vi "Alpha Ver 1.3.vi"() -> ()   [LabVIEW 2015]
uses:
  <instrlib>/Keithley 622x LV 2009/Configure/Source/Typedefs/KE622x -- Current Range.ctl
  <instrlib>/Keithley 622x LV 2009/Configure/Source/Typedefs/KE622x -- Current Ranges.ctl
  <instrlib>/Keithley 622x LV 2009/Typedefs/KE622x -- On Off Control.ctl
  <instrlib>/Keithley 622x LV 2009/Utility/Typedefs/KE622x -- Instrument Type.ctl
  <instrlib>/Keithley 622x LV 2009/Configure/Source/Typedefs/KE622x -- Voltage Limit.ctl
  <instrlib>/Keithley 2000/Public/Configure/Configure DC Volts.vi
  <userlib>/LV-Link3/PolySubVIs/DtCreateAinChan.vi
  <userlib>/LV-Link3/PolySubVIs/DtOLReadMultipleSingle.vi
  <instrlib>/Keithley 2000/Keithley 2000.lvlib
  <instrlib>/Keithley 622x LV 2009/Keithley 622x.lvlib
panel:
  in  "Lock-In, Y":dbl=1.0
  in  "Lock-In, X":dbl=1.0
  in  "DAQ A4":dbl=1.0
  in  "DAQ A3":dbl=1.0
  in  "DAQ A2":dbl=1.0
  in  "DAQ A1":dbl=1.0
  in  "DAQ A0":dbl=1.0
  in  "2000":dbl=1.0
  in  "Current":dbl=1000.0
  in  "Display Type 3":u16(ring)=3 items=["X %", "Y %", "X Calibrated", "Y Calibrated", "Mag %", "Mag Calibrated", "Phase Degrees", "Ratio", "ADC 1", "ADC 2", "ADC 3", "ADC 4 ", "Noise %", "Noise Calibrated", "Ref Frequency", "", ""]
  in  "Display Type 2":u16(ring)=2 items=["X %", "Y %", "X Calibrated", "Y Calibrated", "Mag %", "Mag Calibrated", "Phase Degrees", "Ratio", "ADC 1", "ADC 2", "ADC 3", "ADC 4 ", "Noise %", "Noise Calibrated", "Ref Frequency", "", ""]
  out "Units 3":string
  out "Display 3":dbl format="%.3f"
  out "Units 2":string
  out "Display 2":dbl format="%.3f"
  out "DAQ A4":dbl format="%#_13g"
  out "DAQ_clust":T1
  out "DAQ A3":dbl format="%#_13g"
  out "DAQ A2":dbl format="%#_13g"
  out "DAQ A1":dbl format="%#_13g"
  out "Real stop cur":dbl format="%#_13g"
  out "Real start cur":dbl format="%#_13g"
  in  "Stop cur prefix":u16(ring)=2
  in  "Start cur prefix":u16(ring)=2
  out "MULTIPLE GRAPHS":cluster{dbl[], dbl[]}[](graph)
  in  "X-Axis":T2(ring)
  in  "Range":u8(ring)=20 items=["100nV", "200nV", "500nV", "1µV", "2µV", "5µV", "10µV", "20µV", "50µV", "100µV", "200µV", "500µV", "1mV", "2mV", "5mV", "10mV", "20mV", "50mV", "100mV", "200mV", "500mV", "1V"]
  in  "Display Type copy":u16(ring)=3 items=["X %", "Y %", "X Calibrated", "Y Calibrated", "Mag %", "Mag Calibrated", "Phase Degrees", "Ratio", "ADC 1", "ADC 2", "ADC 3", "ADC 4 ", "Noise %", "Noise Calibrated", "Ref Frequency", "", ""]
  out "Units copy":string
  out "Display copy":dbl format="%.3f"
  out "Overload":bool
  out "Display":dbl format="%.3f"
  out "Units":string
  in  "Display Type":u16(ring)=2 items=["X %", "Y %", "X Calibrated", "Y Calibrated", "Mag %", "Mag Calibrated", "Phase Degrees", "Ratio", "ADC 1", "ADC 2", "ADC 3", "ADC 4 ", "Noise %", "Noise Calibrated", "Ref Frequency", "", ""]
  in  "Time Constant":u16(ring) items=["MIN", "1ms", "3ms", "10ms", "30ms", "100ms", "300ms", "1s", "3s", "10s", "30s", "100s", "300s"]
  in  "Slope":u8(ring) items=["6db/octave", "12dB/octave"]
  in  "Dynamic Reserve":u16(ring) items=["High Stability", "Normal", "High Reserve"]
  in  "Auto Sensitivity":bool
  in  "Auto Measure":bool
  out "6221_error_out":errorcluster
  out "2000_error_out":errorcluster
  out "5110_error_out":errorcluster
  out "Input Mode":i32(ring) items=[" Voltage Input (A or A-B) ", "Current Input 10E6 V/A", "Current Input 10E8 V/A"]
  out "5110":refnum<visa-resource-name>
  in  "GPIB Address":i8=11 min=1 max=32 step=1
  out "DAQ A0":dbl format="%#_13g"
  out "2000":dbl format="%#_13g"
  in  "Device":string(combo)
  in  "Number \nof points":i32
  in  "Folder\nprename":string
  out "TIME GRAPH":cluster{dbl[], dbl[]}[](graph)
  out "T0":u32
  out "LIMIT":bool
  out "LIMIT":bool
  out "Error Code":string
  in  "Comments":string
  out "file":refnum<file>
  out "2000":refnum<visa-resource-name>
  out "6221":refnum<visa-resource-name>
  out "Step  (A)":dbl=5e-05 format="%#_3p"
  in  "Stop\ncurrent (A)":dbl=2.0 format="%#_6p"
  in  "Start \ncurrent (A)":dbl=1.0 format="%#_6p"
  in  "Check For SCPI Errors? (T)":bool=TRUE
  out "Interlock Tripped?":bool
  out "Compliance?":bool
  in  "Turn Off Output \nIf Compliance?":bool=TRUE
  in  "Turning ON/OFF\ncurrent output":T3=enum."On"
  in  "Range Selection":T4={"Auto Range?"=TRUE, "Man / Selected\nRange"=enum."2nA"}
  # "FILE CONFIGURATION"
  # "ADMIN PANEL"
  # "KEITHLEY 6221 CONFIGURATION (ADMIN ONLY)"
  # "KEITHLEY DAQ CONFIGURATION (ADMIN ONLY)"
  # "PRINCETON LOCK-IN AMP (ADMIN ONLY)"
  # "I don't know what the hell it is,\njust don't touch it"
  # "SENSITIVITY"
  # "INPUT CONFIGURATION"
  # "READINGS"
  # "START, STOP, STEP, CONFIGURATION"
  # "IF ON"
  # "Output Channels Time - Constant \nSlope & Dynamic Reserve"
  # "Compliance = Limiting output voltage\nThis switch determines if we want to switch \noff the current output if wee exceed compliance"
  # "LOCK-IN READINGS"
  # "RIGHT DISPLAY"
  # "LEFT DISPLAY"
  # "There is a safe switch at \nthe back of the instrument \nThis indicator shows if it is on"
  # "You have hit a damn jackpot \nby exceeding the limited voltage\nCongrats"
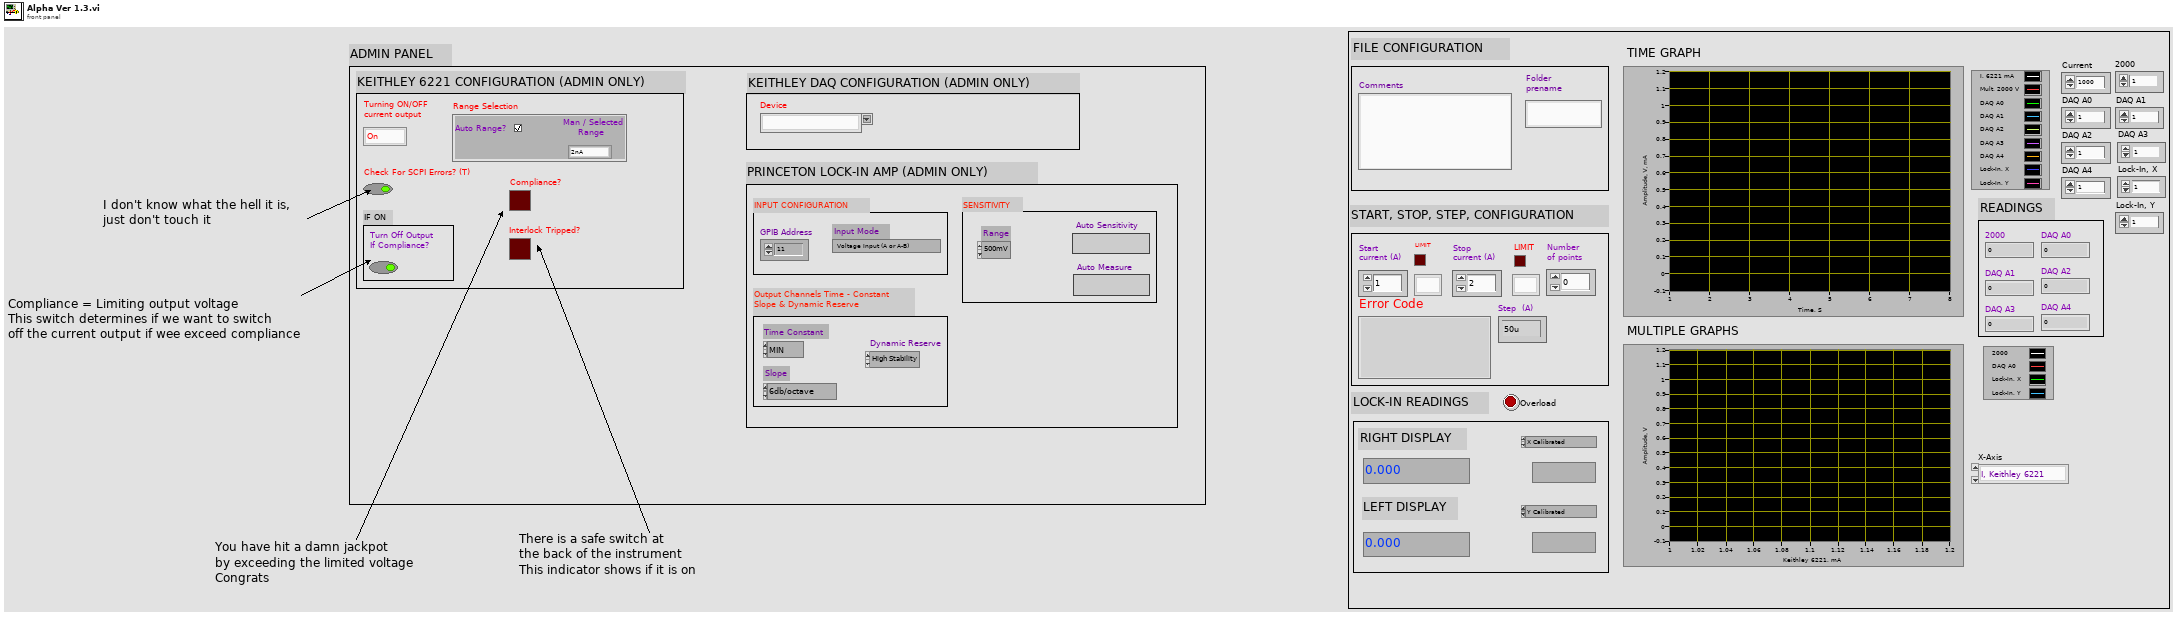
[diagram p1: front panel]
types:
  T1 = cluster{"Task out":i32, "Actual Number of Channels":u32, "error out":errorcluster}
  T2 = enum16{"I, Keithley 6221", "V, Keithley 2000", "V, Keithley DAQ A0", "V, Keithley DAQ A1", "V, Keithley DAQ A2", "V, Keithley DAQ A3", "V, Keithley DAQ A4", "V, Lock-In X", "V, Lock-In Y"}
  T3 = typedef "Keithley 622x.lvlib/KE622x -- On Off Control.ctl" = enum16{"Off", "On"}
  T4 = typedef "Keithley 622x.lvlib/KE622x -- Current Range.ctl" = cluster{"Auto Range?":bool, "Man / Selected\nRange":T5}
  T5 = typedef "Keithley 622x.lvlib/KE622x -- Current Ranges.ctl" = enum16{"2nA", "20nA", "200nA", "2uA", "20uA", "200uA", "2mA", "20mA", "100mA"}
  T6 = typedef "Keithley 622x.lvlib/KE622x -- Instrument Type.ctl" = enum16{"KE6220", "KE6221"}
  T7 = typedef "Keithley 622x.lvlib/KE622x -- Voltage Limit.ctl" = dbl
  T8 = cluster{"Task out":i32, "error out":errorcluster}
  T9 = cluster{dbl, dbl, dbl, dbl, dbl, "Measurement":dbl}
  T10 = cluster{dbl[], dbl[], dbl[], dbl[], dbl[], dbl[], dbl[], dbl[], dbl[], dbl[]}
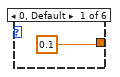
[diagram p2: hidden frame]
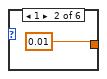
[diagram p3: hidden frame]
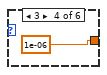
[diagram p4: hidden frame]
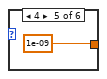
[diagram p5: hidden frame]
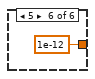
[diagram p6: hidden frame]
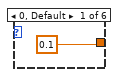
[diagram p7: hidden frame]
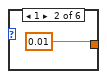
[diagram p8: hidden frame]
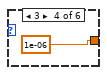
[diagram p9: hidden frame]
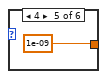
[diagram p10: hidden frame]
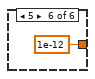
[diagram p11: hidden frame]
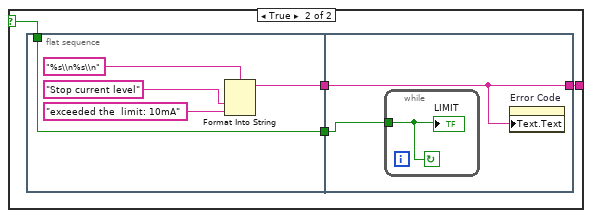
[diagram p12: hidden frame]
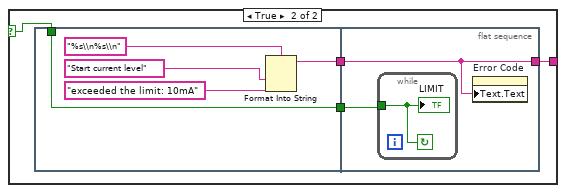
[diagram p13: hidden frame]
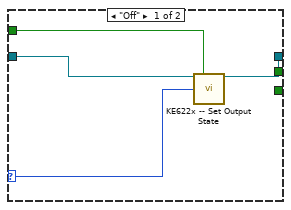
[diagram p14: hidden frame]
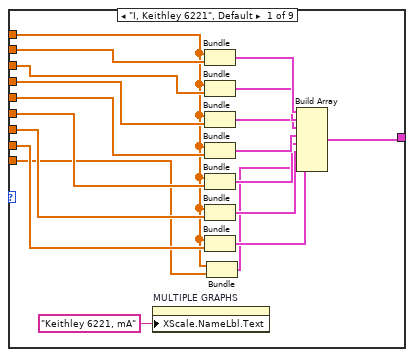
[diagram p15: hidden frame]
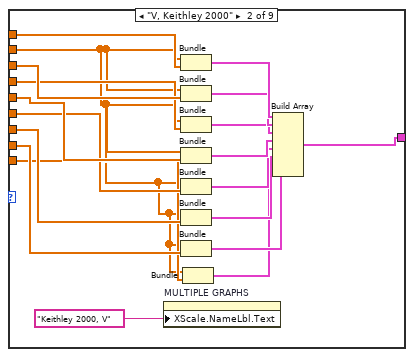
[diagram p16: hidden frame]
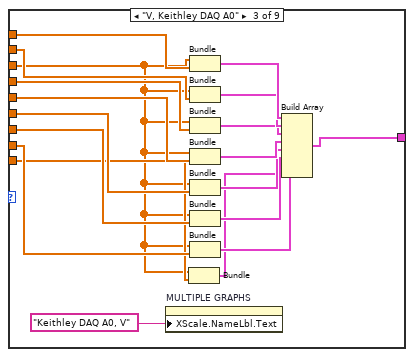
[diagram p17: hidden frame]
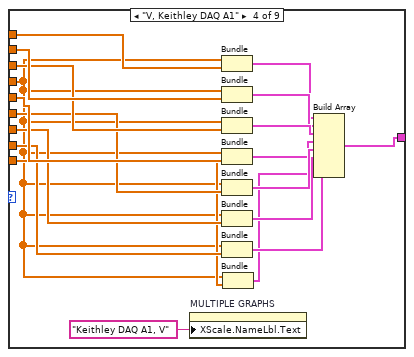
[diagram p18: hidden frame]
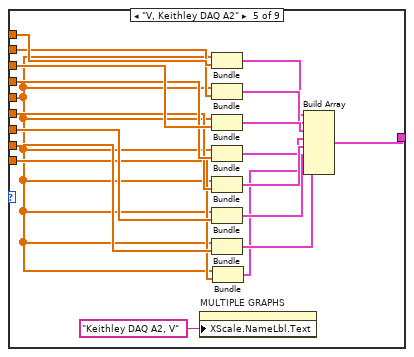
[diagram p19: hidden frame]
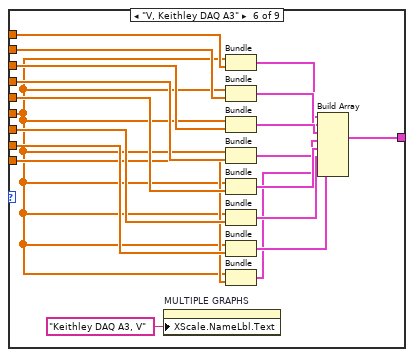
[diagram p20: hidden frame]
diagram:
  n1 = flat-sequence {
    tunnel: [w175] -> w7
    tunnel: [w174] -> w6
    tunnel: [w173] -> w5
    tunnel: [w172] -> w4
    tunnel: [w171] -> w3
    tunnel: [w170] -> w2
    tunnel: [w159] -> w1
    tunnel: w7 -> [w889]
    tunnel: w6 -> [w888]
    tunnel: w5 -> [w887]
    tunnel: w4 -> [w886]
    tunnel: w3 -> [w885]
    tunnel: w2 -> [w884]
    tunnel: w1 -> [w883]
    frame #0 {
      # "File configuration"
      # "Start, Stop, Step"
      # "Time Intit"
      # "Initializing instruments"
      n2 = flat-sequence {
        frame #0 {
          w16 = TRUE  # reset
          w15 = FALSE  # ID query
          # "Initialize Lock-In 5110"
          # "Initialize Keithley 2000"
          # "Initialize Keithley 6221"
          n3 = call <instrlib>:"Initialize.vi"("VISA resource name"=refnum<visa-resource-name> "KEITHLEY_MULTIMETER") -> ("VISA resource name out"=w20:refnum<visa-resource-name>)  [unwired: 17 in, 1 out]
          n4 = call <instrlib>:"Initialize.vi"("VISA resource name"=refnum<visa-resource-name> "KEITHLEY_DC_AC_CURRENT_SOURCE", "Error Queue Option"=enum16{"Clear Error Queue", "Error Query"}."Clear Error Queue", "Instrument Type"=KE622x_--_Instrument_Type."KE6221") -> ("VISA resource name out"=→"6221":refnum<visa-resource-name>, "error out"=→"6221_error_out":errorcluster)  [unwired: 11 in]
          n5 = call "SR51XX Initialize"("VISA session (for class)"=refnum<visa-resource-name> "LOCK_IN_5110_PRINCETON", "Interface"=FALSE, "ID query"=w15, "GPIB Address"="GPIB Address", "reset"=w16) -> ("VISA session"=→"5110":refnum<visa-resource-name>, "error out"=→"5110_error_out":errorcluster)  [unwired: 8 in, 1 out]
          n6 = call-poly <instrlib>:"Configure Measurement.vi"("VISA resource name"=w20) -> ("VISA resource name out"=→"2000":refnum<visa-resource-name>, "error out"=→"2000_error_out":errorcluster)  [unwired: 17 in]
        }
        frame #1 {
          # "Initialize Keithley DAQ \n(getting board name)"
          n7 = call <userlib>:"DtOLGetBoardNames.vi"() -> ("Number of boards"=w25:u32)  [unwired: 9 in, 2 out]
          n8 = Initialize Array("", w25) -> (w27:string[])
          n9 = for {
            N: w25 -> [_]
            shift-right: [w33] -> w30
            shift-left: w27 -> [w34]
            i -> [w32]
            n10 = Add(x=1, y=w32) -> (x+y=w36:i32)
            n11 = call <userlib>:"DtOLGetBoardNames.vi"("Select Board"=w36) -> ("Board Name"=w31:string)  [unwired: 8 in, 2 out]
            n12 = Replace Array Subset(array=w34, new element=w31, index=w32) -> (w33:string[])
          }
          n13 = Index Array(array=w30, index=0) -> (element=w29:string)
          n14 = property on="Device" class="CmbBox"("Strings[]"=w30, "Value"=w29) -> ()  [unwired: 2 in, 2 out]
        }
        frame #2 {
          # "Calculating steps by number\nof points"
          # "Putting in a loop \ninstead of \"STOP\""
          n15 = local read "Real stop cur"() -> (w53:dbl)
          n16 = local read "Real start cur"() -> (w54:dbl)
          n17 = case shown="2" "Start cur prefix" {
            tunnel: [0.1 0.01 0.001 1e-06 1e-09 1e-12] -> w42
            frame 0, Default {
            }
            frame 1 {
            }
            frame 2 {
            }
            frame 3 {
            }
            frame 4 {
            }
            frame 5 {
            }
          }
          n18 = case shown="2" "Stop cur prefix" {
            tunnel: [0.1 0.01 0.001 1e-06 1e-09 1e-12] -> w40
            frame 0, Default {
            }
            frame 1 {
            }
            frame 2 {
            }
            frame 3 {
            }
            frame 4 {
            }
            frame 5 {
            }
          }
          n19 = Subtract(x=w53, y=w54) -> (x-y=w56:dbl)
          n20 = Multiply(x=w42, y="Start \ncurrent (A)") -> (x*y=w38:dbl)
          "Real start cur" <- w38
          n21 = Divide(x=w56, y="Number \nof points") -> (x/y=→"Step  (A)":dbl)
          n22 = Multiply(x=w40, y="Stop\ncurrent (A)") -> (x*y=w37:dbl)
          "Real stop cur" <- w37
          n23 = Greater?(x=w37, y=T7 0.01) -> (0:w48:bool)
          n24 = Greater?(x=w38, y=T7 0.01) -> (0:w47:bool)
          n25 = case shown="False" w48 {
            selector: w48 -> [_ w72]
            tunnel: [w69 w75] -> w50
            frame False {
              n26 = Format Into String(format string="%s\\n", "Start current level is OK" ("false string")) -> (resulting string=w69:string)  [unwired: 2 in, 1 out]
            }
            frame True {
              n27 = flat-sequence {
                tunnel: [w77] -> w74
                tunnel: [w76] -> w73
                tunnel: w72 -> [w76]
                tunnel: [w81] -> w75
                tunnel: w74 -> [w81]
                tunnel: w73 -> [w82]
                frame #0 {
                  n28 = Format Into String(format string="%s\\n%s\\n", "Stop current level" ("String"), "exceeded the  limit: 10mA" ("input 2")) -> (resulting string=w77:string)  [unwired: 2 in, 1 out]
                }
                frame #1 {
                  n29 = while {
                    tunnel: w82 -> [w83]
                    stop <- w83 continue-if-true
                    "LIMIT" <- w83
                  }
                  n30 = property on="Error Code" class="Str"("Text.Text"=w81) -> ()  [unwired: 2 in, 2 out]
                }
              }
            }
          }
          n31 = case shown="False" w47 {
            selector: w47 -> [_ w88]
            tunnel: [w84 w90] -> w49
            frame False {
              n32 = Format Into String(format string="%s\\n", "Start current level is OK" ("false string")) -> (resulting string=w84:string)  [unwired: 2 in, 1 out]
            }
            frame True {
              n33 = flat-sequence {
                tunnel: [w92] -> w89
                tunnel: w88 -> [w91]
                tunnel: [w91] -> w87
                tunnel: [w96] -> w90
                tunnel: w89 -> [w96]
                tunnel: w87 -> [w97]
                frame #0 {
                  n34 = Format Into String(format string="%s\\n%s\\n", "Start current level" ("String"), "exceeded the limit: 10mA" ("input 2")) -> (resulting string=w92:string)  [unwired: 2 in, 1 out]
                }
                frame #1 {
                  n35 = while {
                    tunnel: w97 -> [w98]
                    stop <- w98 continue-if-true
                    "LIMIT" <- w98
                  }
                  n36 = property on="Error Code" class="Str"("Text.Text"=w96) -> ()  [unwired: 2 in, 2 out]
                }
              }
            }
          }
          n37 = Concatenate Strings(w49, w50) -> (→"Error Code":string)
        }
        frame #3 {
          n38 = flat-sequence {
            frame #0 {
              # "Creating folder&file"
              n39 = call "folder_creation.vi"("Name"="Folder\nprename") -> ("String"=w100:string)
              n40 = call "file_creation.vi"("String"=w100) -> ("refnum out"=→"file":refnum<file>)
            }
            frame #1 {
              # "Creating comments"
              n41 = local read "file"() -> (w102:refnum<file>)
              n42 = Format Into String(format string="# %s\\n", initial string=w102, "Comments") -> ()  [unwired: 1 in, 2 out]
            }
            frame #2 {
              # "Writing instr params"
              n43 = local read "5110"() -> (w110:refnum<visa-resource-name>)
              n44 = local read "Real stop cur"() -> (w108:dbl)
              n45 = local read "file"() -> (w105:refnum<file>)
              n46 = local read "Real start cur"() -> (w109:dbl)
              n47 = call "com_inst.vi"("Stop current"=w108, "Start current"=w109, "VISA session (for class)"=w110) -> ("concatenated string"=w106:string)
              n48 = Format Into String(format string="# %s\\n", initial string=w105, w106) -> ()  [unwired: 1 in, 2 out]
            }
            frame #3 {
              # "Adding headlines"
              n49 = local read "file"() -> (w122:refnum<file>)
              n50 = Format Into String(format string="# %-6s  %-12s %-12s %-14s %-12s %-14s %-12s %-12s %-14s%-14s\\n", initial string=w122, "t, s" ("input 3"), "2000, V" ("input 1"), "DAQ A0, V" ("input 2"), "DAQ A1, V" ("input 2"), "DAQ A2, V" ("input 2"), "DAQ A3, V" ("input 2"), "DAQ A4, V" ("input 2"), "5110_X, V" ("input 3"), "5110_Y, V " ("input 3"), "6221, A" ("input 3")) -> ()  [unwired: 1 in, 2 out]
            }
          }
        }
      }
      n51 = Tick Count (ms)() -> (millisecond timer value=→"T0":u32)
    }
    frame #1 {
      # "Configuring Keithley DAQ just before measuments"
      # "Configuring Keithley 6221 just before measuments"
      n52 = flat-sequence {
        tunnel: [w133] -> w123
        tunnel: [w151] -> _
        tunnel: [w153] -> _
        tunnel: w123 -> [w152]
        frame #0 {
          # "Current range \nselection check"
          # "Checking for compliance\nand interlock errors"
          n53 = local read "6221"() -> (w136:refnum<visa-resource-name>)
          n54 = call <instrlib>:"KE622x -- Set Current Range.vi"("Resource In"=w136, "Current Range In"="Range Selection", "Read Back Set Values? (T)"=FALSE) -> ("Resource Out (dupl)"=w141:refnum<visa-resource-name>)  [unwired: 10 in, 2 out]
          n55 = case shown="\"On\"" "Turning ON/OFF\ncurrent output" {
            selector: "Turning ON/OFF\ncurrent output" -> [w145 _]
            tunnel: [_ w149] -> w139
            tunnel: [_ w148] -> w140
            tunnel: "Check For SCPI Errors? (T)" -> [w144 _]
            tunnel: w141 -> [w142 w147]
            tunnel: [w143 w146] -> w133
            frame "Off" {
              n56 = call <instrlib>:"KE622x -- Set Output State.vi"("Resource In"=w142, "Check For SCPI Errors? (T)"=w144, "Output State"=w145) -> ("Resource Out (dupl)"=w143:refnum<visa-resource-name>)  [unwired: 11 in, 1 out]
            }
            frame "On" {
              n57 = call <instrlib>:"KE622x -- Turn Output On And Check For Errors.vi"("Resource In"=w147, "Turn Off Output If Compliance?"="Turn Off Output \nIf Compliance?") -> ("Resource Out (dupl)"=w146:refnum<visa-resource-name>, "Interlock Tripped?"=w149:bool, "Compliance?"=w148:bool)  [unwired: 10 in, 1 out]
            }
          }
          "Interlock Tripped?" <- w139
          "Compliance?" <- w140
        }
        frame #1 {
          # "Setting start current"
          n58 = local read "Real start cur"() -> (w151:dbl)
          n59 = Wait (ms)(milliseconds to wait=u32 100) -> ()  [unwired: 1 out]
          n60 = call <instrlib>:"KE622x -- Set Current Level.vi"("Resource In"=w152, "Current Level (A) In"=w151) -> ("Resource Out (dupl)"=w153:refnum<visa-resource-name>)  [unwired: 12 in, 1 out]
        }
      }
      n61 = flat-sequence {
        frame #0 {
          w128 = 100 items=["SingleEnded"=100, "Differential"=101] ("Channel Type")
          # "Configure the input channel"
          n62 = call-poly <userlib>:"DtOLCreateTask.vi"("Channel Type"=w128, "Range Min"=-10.0, "Range Max"=10.0, "Board Name"="Device", "Channel"="0:4" ("Channels")) -> ("Task out"=w127:i32, "Actual Number of Channels"=w126:u32, "error out"=w125:errorcluster)  [unwired: 8 in]
          n63 = Bundle("Task out"=w127, "Actual Number of Channels"=w126, "error out"=w125) -> (→"DAQ_clust":T1)  [unwired: 1 in]
        }
      }
    }
    frame #2 {
      n64 = local read "5110"() -> (w166:refnum<visa-resource-name>)
      n65 = local read "2000"() -> (w165:refnum<visa-resource-name>)
      n66 = local read "6221"() -> (w164:refnum<visa-resource-name>)
      n67 = local read "5110_error_out"() -> (w163:errorcluster)
      n68 = local read "6221_error_out"() -> (w162:errorcluster)
      n69 = local read "2000_error_out"() -> (w161:errorcluster)
      n70 = local read "DAQ_clust"() -> (w160:T1)
      n71 = while {
        shift-right: [w320] -> _
        shift-left: dbl[] [] -> [w453]
        shift-right: [w321] -> _
        shift-left: i32[] [] -> [w452]
        tunnel: w165 -> [w450]
        tunnel: w164 -> [w449]
        shift-right: [w273] -> _
        shift-left: dbl[] [] -> [w442]
        tunnel: [w441] -> w175
        tunnel: [w440] -> w174
        tunnel: [w438] -> w173
        tunnel: [w435] -> w172
        tunnel: w166 -> [w432]
        tunnel: w163 -> [w431]
        tunnel: w162 -> [w423]
        tunnel: w161 -> [w422]
        tunnel: [w385] -> w171
        tunnel: [w382] -> w170
        shift-right: [w275] -> _
        shift-left: dbl[] [] -> [w381]
        shift-right: [w276] -> _
        shift-left: dbl[] [] -> [w380]
        shift-right: [w322] -> _
        shift-left: dbl[] [] -> [w377]
        tunnel: w160 -> [w335]
        tunnel: [w334] -> w159
        shift-right: [w319] -> _
        shift-left: dbl[] [] -> [w333]
        shift-right: [w318] -> _
        shift-left: dbl[] [] -> [w332]
        shift-right: [w317] -> _
        shift-left: dbl[] [] -> [w331]
        shift-right: [w274] -> _
        shift-left: dbl[] [] -> [w278]
        i -> [w424]
        stop <- w443 stop-if-true
        # "V, DAQ A4"
        # "V, DAQ A3"
        # "V, DAQ A2"
        # "V, DAQ A1"
        # "Y-V, 5110"
        # "X-V, 5110"
        # "I, 6221"
        # "Config delay"
        # "Control subVI 5110"
        # "Read config 5110"
        # "Measurement config 5110"
        # "Time config 5110"
        # "Configuring Right Display 5110"
        # "Configuring Left Display 5110"
        # "Setting 6221 current"
        # "Delay before measuremens"
        # "Getting the data from DAQ and 2000"
        # "Changing input current"
        # "Time"
        # "V, DAQ A0"
        # "V, 2000"
        n72 = local read "T0"() -> (w451:u32)
        n73 = Quotient & Remainder(x=w424, y=10) -> (floor(x/y)=w429:i32)  [unwired: 1 out]
        n74 = Equal?(x=0, y=w424) -> (x = y?=w426:bool)
        n75 = Subtract(x=w413, y=w451) -> (x-y=w345:u32)
        n76 = Equal?(x=1, y=w429) -> (x = y?=w425:bool)
        n77 = flat-sequence {
          tunnel: w450 -> [w635]
          tunnel: [w635] -> w376
          tunnel: w449 -> [w634]
          tunnel: [w634] -> w374
          tunnel: w432 -> [w632]
          tunnel: [w632] -> w372
          tunnel: [w631] -> w370
          tunnel: w431 -> [w631]
          tunnel: w426 -> [w630]
          tunnel: [w630] -> w368
          tunnel: w425 -> [w629]
          tunnel: [w629] -> w366
          tunnel: w423 -> [w628]
          tunnel: [w628] -> w364
          tunnel: w422 -> [w627]
          tunnel: [w627] -> w362
          tunnel: [w626] -> w413
          tunnel: [w625] -> w336
          tunnel: w335 -> [w625]
          tunnel: w376 -> [w650]
          tunnel: [w650] -> w375
          tunnel: w374 -> [w649]
          tunnel: [w649] -> w373
          tunnel: w372 -> [w648]
          tunnel: [w648] -> w371
          tunnel: w370 -> [w647]
          tunnel: [w647] -> w369
          tunnel: w368 -> [w646]
          tunnel: [w646] -> w367
          tunnel: w366 -> [w645]
          tunnel: [w645] -> w365
          tunnel: w364 -> [w644]
          tunnel: [w644] -> w363
          tunnel: w362 -> [w643]
          tunnel: [w643] -> w361
          tunnel: [w636] -> w337
          tunnel: w336 -> [w636]
          tunnel: w375 -> [w663]
          tunnel: [w663] -> w412
          tunnel: w373 -> [w662]
          tunnel: [w662] -> w411
          tunnel: w371 -> [w661]
          tunnel: w369 -> [w658]
          tunnel: [w657] -> w410
          tunnel: [w656] -> w409
          tunnel: w367 -> [w655]
          tunnel: [w655] -> w408
          tunnel: w365 -> [w654]
          tunnel: w363 -> [w653]
          tunnel: [w653] -> w407
          tunnel: w361 -> [w652]
          tunnel: [w652] -> w406
          tunnel: [w651] -> w338
          tunnel: w337 -> [w651]
          tunnel: w412 -> [w688]
          tunnel: [w688] -> w405
          tunnel: w411 -> [w687]
          tunnel: [w687] -> w404
          tunnel: w410 -> [w684]
          tunnel: [w683] -> w403
          tunnel: w409 -> [w682]
          tunnel: [w681] -> w402
          tunnel: w408 -> [w679]
          tunnel: [w679] -> w401
          tunnel: w407 -> [w686]
          tunnel: [w686] -> w400
          tunnel: w406 -> [w685]
          tunnel: [w685] -> w399
          tunnel: ["Auto Measure"] -> w398
          tunnel: ["Auto Sensitivity"] -> w397
          tunnel: [w674] -> w396
          tunnel: [w671] -> w339
          tunnel: w338 -> [w671]
          tunnel: w405 -> [w707]
          tunnel: [w707] -> w360
          tunnel: w404 -> [w706]
          tunnel: [w706] -> w359
          tunnel: w403 -> [w699]
          tunnel: w402 -> [w697]
          tunnel: [w696] -> w358
          tunnel: w401 -> [w703]
          tunnel: [w703] -> w357
          tunnel: w400 -> [w705]
          tunnel: [w705] -> w356
          tunnel: w399 -> [w704]
          tunnel: [w704] -> w355
          tunnel: w398 -> [w701]
          tunnel: [w701] -> w354
          tunnel: w397 -> [w702]
          tunnel: [w702] -> w353
          tunnel: w396 -> [w692]
          tunnel: [w692] -> w352
          tunnel: [w698] -> w351
          tunnel: ["Time Constant"] -> w350
          tunnel: ["Slope"] -> w349
          tunnel: [w689] -> w340
          tunnel: w339 -> [w689]
          tunnel: [w729] -> w270
          tunnel: [w728] -> w269
          tunnel: [w714] -> w268
          tunnel: [w727] -> w267
          tunnel: [w726] -> w266
          tunnel: [w725] -> w265
          tunnel: [w724] -> w264
          tunnel: [w723] -> w263
          tunnel: [w716] -> w262
          tunnel: [w719] -> w261
          tunnel: [w717] -> w260
          tunnel: [w722] -> w259
          tunnel: w349 -> [w722]
          tunnel: w350 -> [w717]
          tunnel: w351 -> [w720]
          tunnel: w352 -> [w716]
          tunnel: w353 -> [w723]
          tunnel: w354 -> [w724]
          tunnel: w355 -> [w725]
          tunnel: w356 -> [w726]
          tunnel: w357 -> [w727]
          tunnel: w358 -> [w715]
          tunnel: w359 -> [w728]
          tunnel: w360 -> [w729]
          tunnel: [w708] -> w258
          tunnel: w340 -> [w708]
          tunnel: w270 -> [w752]
          tunnel: [w752] -> w257
          tunnel: w269 -> [w751]
          tunnel: [w751] -> w255
          tunnel: w268 -> [w743]
          tunnel: [w742] -> w253
          tunnel: w267 -> [w750]
          tunnel: [w750] -> w251
          tunnel: w266 -> [w749]
          tunnel: [w749] -> w249
          tunnel: w265 -> [w748]
          tunnel: [w748] -> w247
          tunnel: w264 -> [w747]
          tunnel: [w747] -> w245
          tunnel: w263 -> [w746]
          tunnel: [w746] -> w243
          tunnel: w262 -> [w737]
          tunnel: [w737] -> w241
          tunnel: w261 -> [w744]
          tunnel: [w741] -> w239
          tunnel: w260 -> [w739]
          tunnel: [w739] -> w237
          tunnel: w259 -> [w736]
          tunnel: [w736] -> w235
          tunnel: w258 -> [w745]
          tunnel: [w745] -> w233
          tunnel: [w732] -> w230
          tunnel: w257 -> [w775]
          tunnel: [w775] -> w256
          tunnel: w255 -> [w774]
          tunnel: [w774] -> w254
          tunnel: w253 -> [w765]
          tunnel: [w764] -> w252
          tunnel: w251 -> [w773]
          tunnel: [w773] -> w250
          tunnel: w249 -> [w772]
          tunnel: [w772] -> w248
          tunnel: w247 -> [w771]
          tunnel: [w771] -> w246
          tunnel: w245 -> [w770]
          tunnel: [w770] -> w244
          tunnel: w243 -> [w769]
          tunnel: [w769] -> w242
          tunnel: w241 -> [w760]
          tunnel: [w760] -> w240
          tunnel: w239 -> [w767]
          tunnel: [w766] -> w238
          tunnel: w237 -> [w762]
          tunnel: [w762] -> w236
          tunnel: w235 -> [w759]
          tunnel: [w759] -> w234
          tunnel: w233 -> [w768]
          tunnel: [w768] -> w232
          tunnel: [w755] -> w231
          tunnel: w256 -> [w797]
          tunnel: [w797] -> w395
          tunnel: w254 -> [w796]
          tunnel: [w796] -> w394
          tunnel: w252 -> [w783]
          tunnel: w250 -> [w795]
          tunnel: [w795] -> w393
          tunnel: w248 -> [w794]
          tunnel: [w794] -> w392
          tunnel: w246 -> [w793]
          tunnel: [w793] -> w391
          tunnel: w244 -> [w792]
          tunnel: [w792] -> w390
          tunnel: w242 -> [w791]
          tunnel: [w791] -> w389
          tunnel: w240 -> [w784]
          tunnel: w238 -> [w781]
          tunnel: [w780] -> w388
          tunnel: w236 -> [w785]
          tunnel: w234 -> [w786]
          tunnel: [w782] -> w387
          tunnel: [w779] -> w386
          tunnel: [w776] -> w341
          tunnel: w232 -> [w776]
          tunnel: [w801] -> w447
          tunnel: w424 -> [w809]
          tunnel: [w805] -> w443
          tunnel: [w799] -> w445
          tunnel: [w807] -> w444
          tunnel: [w804] -> w421
          tunnel: [w803] -> w420
          tunnel: [w802] -> w419
          tunnel: [w800] -> w418
          tunnel: [w799] -> w330
          tunnel: w386 -> [_]
          tunnel: w387 -> [w802]
          tunnel: w388 -> [w800]
          tunnel: w389 -> [_]
          tunnel: w390 -> [_]
          tunnel: w391 -> [w804]
          tunnel: w392 -> [w803]
          tunnel: w393 -> [_]
          tunnel: w394 -> [w807]
          tunnel: w395 -> [w801]
          tunnel: [w798] -> w342
          tunnel: w341 -> [w798]
          tunnel: w447 -> [w821]
          tunnel: [w821] -> w446
          tunnel: w445 -> [w820]
          tunnel: w444 -> [w819]
          tunnel: [w818] -> w439
          tunnel: [w817] -> w436
          tunnel: w421 -> [w815]
          tunnel: w420 -> [w816]
          tunnel: w419 -> [w813]
          tunnel: w418 -> [w814]
          tunnel: [w815] -> w417
          tunnel: [w814] -> w414
          tunnel: [w813] -> w383
          tunnel: [w812] -> w343
          tunnel: w342 -> [w812]
          tunnel: w446 -> [w829]
          tunnel: [w829] -> w448
          tunnel: w439 -> [w827]
          tunnel: [w827] -> w437
          tunnel: w436 -> [w826]
          tunnel: [w826] -> w434
          tunnel: w417 -> [w825]
          tunnel: [w825] -> w416
          tunnel: [w824] -> w415
          tunnel: w414 -> [w824]
          tunnel: [w823] -> w384
          tunnel: w383 -> [w823]
          tunnel: [w822] -> w344
          tunnel: w343 -> [w822]
          tunnel: [w866] -> w303
          tunnel: [w833] -> w302
          tunnel: [w865] -> w301
          tunnel: [w864] -> w300
          tunnel: [w863] -> w299
          tunnel: [w862] -> w298
          tunnel: [w834] -> w297
          tunnel: [w866] -> w296
          tunnel: [w861] -> w295
          tunnel: [w860] -> w294
          tunnel: [w859] -> w293
          tunnel: w344 -> [w856]
          tunnel: w384 -> [w860]
          tunnel: w415 -> [w861]
          tunnel: w416 -> [w857]
          tunnel: w434 -> [w862]
          tunnel: w437 -> [w863]
          tunnel: w448 -> [w858]
          tunnel: [w832] -> w292
          tunnel: [w831] -> w291
          tunnel: [w830] -> w290
          tunnel: [w870] -> w334
          tunnel: [w871] -> w382
          tunnel: [w872] -> w385
          tunnel: [w873] -> w433
          tunnel: [w874] -> w289
          tunnel: [w875] -> w435
          tunnel: [w876] -> w438
          tunnel: [w877] -> w440
          tunnel: [w878] -> w441
          tunnel: [w879] -> w288
          tunnel: [w880] -> w281
          tunnel: w303 -> [w880]
          tunnel: w302 -> [w879]
          tunnel: w301 -> [w878]
          tunnel: w300 -> [w877]
          tunnel: w299 -> [w876]
          tunnel: w298 -> [w875]
          tunnel: w297 -> [w874]
          tunnel: w296 -> [w873]
          tunnel: w295 -> [w872]
          tunnel: w294 -> [w871]
          tunnel: w293 -> [w870]
          tunnel: [w869] -> w287
          tunnel: w292 -> [w869]
          tunnel: [w868] -> w286
          tunnel: w291 -> [w868]
          tunnel: w290 -> [w867]
          tunnel: [w867] -> w282
          frame #0 {
            n78 = Wait Until Next ms Multiple(millisecond multiple=u32 500) -> (millisecond timer value=w626:u32)
          }
          frame #1 {
            n79 = control-ref of="Range"() -> (w642:refnum<vi>)
            n80 = control-ref of="Auto Sensitivity"() -> (w641:refnum<vi>)
            n81 = control-ref of="Auto Measure"() -> (w640:refnum<vi>)
            n82 = control-ref of="Time Constant"() -> (w637:refnum<vi>)
            n83 = control-ref of="Slope"() -> (w638:refnum<vi>)
            n84 = control-ref of="Dynamic Reserve"() -> (w639:refnum<vi>)
            n85 = call "cont_ver_1.0.vi"("Dynamic Reserve"=w639, "Slope"=w638, "Time Constant"=w637, "Auto Measure"=w640, "Auto Sensitivity"=w641, "Range"=w642) -> ()
          }
          frame #2 {
            n86 = case shown="False" w654 {
              tunnel: w661 -> [w665 w670]
              tunnel: [w664 w668] -> w660
              tunnel: [w665 w667] -> w659
              tunnel: w658 -> [w664 w666]
              frame False {
              }
              frame True {
                n87 = call "SR51XX Read Preamp Input Mode"("VISA session (for class)"=w670, "error in (no error)"=w666) -> ("VISA session"=w667:refnum<visa-resource-name>, "Input Mode"=w669:i32, "error out"=w668:errorcluster)  [unwired: 15 in]
                n88 = local write "Input Mode"(w669) -> ()
              }
            }
            n89 = call "SR51XX Configure Signal Channel Input"("VISA session (for class)"=w659, "error in (no error)"=w660, "Update"=w655) -> ("VISA session"=w657:refnum<visa-resource-name>, "error out"=w656:errorcluster)  [unwired: 15 in]
          }
          frame #3 {
            n90 = local read "Input Mode"() -> (w680:i32)
            n91 = call "SR51XX Configure Sensitivity"("VISA session (for class)"=w684, "Input Mode"=w680, "Range"="Range", "error in (no error)"=w682, "Auto Sensitivity"="Auto Sensitivity", "Auto Measure"="Auto Measure", "Update"=w679) -> ("Range Annotations Out[]"=w672:string[], "VISA session"=w683:refnum<visa-resource-name>, "Auto Sensitivity out"=w676:bool, "Auto Measure out"=w675:bool, "Range Out"=w674:u8, "error out"=w681:errorcluster)  [unwired: 7 in]
            n92 = property on="Range" class="Ring (strict)"("Strings []"=w672) -> ()  [unwired: 2 in, 2 out]
            n93 = local write "Auto Sensitivity"(w676) -> ()
            n94 = local write "Auto Measure"(w675) -> ()
            n95 = local write "Range"(w674) -> ()
          }
          frame #4 {
            n96 = Or(x=w702, y=w701) -> (x .or. y?=w700:bool)
            n97 = call "SR51XX Configure Output Channels - Slope, TC and Dyn Reserve"("VISA session (for class)"=w699, "Time Constant"="Time Constant", "Slope"="Slope", "Check TC"=w700, "Dynamic Reserve"="Dynamic Reserve", "error in (no error)"=w697, "Range"=w692, "Update"=w703) -> ("VISA session"=w698:refnum<visa-resource-name>, "Slope Out"=w693:u8, "Time Constant Out"=w694:u16, "error out"=w696:errorcluster)  [unwired: 8 in]
            n98 = local write "Slope"(w693) -> ()
            n99 = local write "Time Constant"(w694) -> ()
          }
          frame #5 {
            n100 = local read "Input Mode"() -> (w721:i32)
            n101 = call "SR5110 Read Output"("VISA session (for class)"=w720, "Input Mode"=w721, "Time Constant"=w717, "Display Type"="Display Type", "Range"=w716, "error in (no error)"=w715, "Slope"=w722) -> ("Units"=→"Units":string, "Display Precision"=w713:i32, "Display"=→"Display":dbl, "VISA session"=w719:refnum<visa-resource-name>, "Available Display Types Out"=w712:string[], "Overload"=→"Overload":bool, "error out"=w714:errorcluster)  [unwired: 4 in, 2 out]
            n102 = property on="Display Type" class="Ring (strict)"("Strings []"=w712) -> ()  [unwired: 2 in, 2 out]
            n103 = property on="Display" class="DigNum (strict)"("Precision"=w713) -> ()  [unwired: 2 in, 2 out]
          }
          frame #6 {
            n104 = local read "Input Mode"() -> (w740:i32)
            n105 = call "SR5110 Read Output"("VISA session (for class)"=w744, "Input Mode"=w740, "Time Constant"=w739, "Display Type"="Display Type 2", "Range"=w737, "error in (no error)"=w743, "Slope"=w736) -> ("Units"=w730:string, "Display Precision"=w734:i32, "Display"=w731:dbl, "VISA session"=w741:refnum<visa-resource-name>, "Available Display Types Out"=w735:string[], "error out"=w742:errorcluster)  [unwired: 4 in, 3 out]
            "Display 2" <- w731
            "Units 2" <- w730
            n106 = call "pref_to_num.vi"("string"=w730) -> ("Numeric"=w733:dbl)
            n107 = property on="Display Type 2" class="Ring (strict)"("Strings []"=w735) -> ()  [unwired: 2 in, 2 out]
            n108 = property on="Display 2" class="DigNum (strict)"("Precision"=w734) -> ()  [unwired: 2 in, 2 out]
            n109 = Multiply(x=w733, y=w731) -> (x*y=w732:dbl)
          }
          frame #7 {
            n110 = local read "Input Mode"() -> (w763:i32)
            n111 = call "SR5110 Read Output"("VISA session (for class)"=w767, "Input Mode"=w763, "Time Constant"=w762, "Display Type"="Display Type 3", "Range"=w760, "error in (no error)"=w765, "Slope"=w759) -> ("Units"=w754:string, "Display Precision"=w758:i32, "Display"=w753:dbl, "VISA session"=w766:refnum<visa-resource-name>, "Available Display Types Out"=w757:string[], "error out"=w764:errorcluster)  [unwired: 4 in, 3 out]
            "Display 3" <- w753
            "Units 3" <- w754
            n112 = property on="Display 3" class="DigNum (strict)"("Precision"=w758) -> ()  [unwired: 2 in, 2 out]
            n113 = call "pref_to_num.vi"("string"=w754) -> ("Numeric"=w756:dbl)
            n114 = property on="Display Type 3" class="Ring (strict)"("Strings []"=w757) -> ()  [unwired: 2 in, 2 out]
            n115 = Multiply(x=w756, y=w753) -> (x*y=w755:dbl)
          }
          frame #8 {
            n116 = local read "Input Mode"() -> (w790:i32)
            n117 = call "SR5110 Read Output"("VISA session (for class)"=w781, "Input Mode"=w790, "Time Constant"=w785, "Display Type"="Display Type copy", "Range"=w784, "error in (no error)"=w783, "Slope"=w786) -> ("Units"=→"Units copy":string, "Display Precision"=w787:i32, "Display"=→"Display copy":dbl, "VISA session"=w780:refnum<visa-resource-name>, "Reference Unlock"=w779:bool, "Available Display Types Out"=w788:string[], "error out"=w782:errorcluster)  [unwired: 4 in, 2 out]
            n118 = property on="Display Type copy" class="Ring (strict)"("Strings []"=w788) -> ()  [unwired: 2 in, 2 out]
            n119 = property on="Display copy" class="DigNum (strict)"("Precision"=w787) -> ()  [unwired: 2 in, 2 out]
          }
          frame #9 {
            n120 = local read "Step  (A)"() -> (w810:dbl)
            n121 = local read "Real start cur"() -> (w811:dbl)
            n122 = Multiply(x=w810, y=w809) -> (x*y=w808:dbl)
            n123 = Add(x=w811, y=w808) -> (x+y=w799:dbl)
            n124 = local read "Real stop cur"() -> (w806:dbl)
            n125 = Greater Or Equal?(x=w799, y=w806) -> (x >= y?=w805:bool)
          }
          frame #10 {
            n126 = call <instrlib>:"KE622x -- Set Current Level.vi"("Resource In"=w819, "Current Level (A) In"=w820, "error in (no error)"=w816) -> ("Resource Out (dupl)"=w817:refnum<visa-resource-name>, "error out"=w818:errorcluster)  [unwired: 11 in]
          }
          frame #11 {
            n127 = Wait Until Next ms Multiple(millisecond multiple=u32 50) -> ()  [unwired: 1 out]
          }
          frame #12 {
            n128 = Unbundle(w856) -> ("Task out"=w855:i32, "Actual Number of Channels"=w853:u32, "error out"=w854:errorcluster)
            n129 = call <instrlib>:"Data Read Single.vi"("VISA resource name"=w858, "error in (no error)"=w857) -> ("VISA resource name out"=w864:refnum<visa-resource-name>, "Measurement"=w866:dbl, "error out"=w865:errorcluster)  [unwired: 13 in, 2 out]
            n130 = call-poly <userlib>:"DtOLRead.vi"("Number Chan to Read"=w853, "error in (no error)"=w854, "Task in"=w855) -> ("error out"=w851:errorcluster, "2D Data out"=w850:dbl[][], "Task out"=w852:i32)  [unwired: 4 in, 2 out]
            n131 = Index Array(array=w850, index (row) #1=0 ("index (row)"), index (row) #2=1 ("index (row)"), index (row) #3=2 ("index (row)"), index (row) #4=3 ("index (row)"), index (row) #5=4 ("index (row)")) -> (element #1=w849:dbl[], element #2=w843:dbl[], element #3=w842:dbl[], element #4=w841:dbl[], element #5=w840:dbl[])  [unwired: 5 in]
            n132 = Index Array(array=w840, index=0) -> (element=w830:dbl)
            n133 = Index Array(array=w849, index=0) -> (element=w834:dbl)
            n134 = Index Array(array=w843, index=0) -> (element=w833:dbl)
            n135 = Index Array(array=w842, index=0) -> (element=w832:dbl)
            n136 = Index Array(array=w841, index=0) -> (element=w831:dbl)
            n137 = Bundle("Task out"=w852, "error out"=w851) -> (w859:T8)  [unwired: 1 in]
          }
          frame #13 {
          }
        }
        n138 = Divide(x=w345, y=u32 1000) -> (x/y=w346:dbl)
        n139 = local read "file"() -> (w348:refnum<file>)
        n140 = Build Array (concatenate)(w452, w346) -> (w328:dbl[])
        n141 = Bundle(w330, w230, w231) -> (w183:cluster{dbl, dbl, dbl})  [unwired: 1 in]
        n142 = Unbundle(w183) -> (w227:dbl, w193:dbl, w188:dbl)
        n143 = Unbundle(w183) -> (w180:dbl, w182:dbl, w181:dbl)
        n144 = Multiply(x=w227, y="Current") -> (x*y=w226:dbl)
        n145 = Multiply(x=w188, y="Lock-In, Y") -> (x*y=w189:dbl)
        n146 = Multiply(x=w193, y="Lock-In, X") -> (x*y=w194:dbl)
        n147 = Build Array (concatenate)(w377, w226) -> (w329:dbl[])
        n148 = Build Array (concatenate)(w381, w194) -> (w280:dbl[])
        n149 = Build Array (concatenate)(w380, w189) -> (w279:dbl[])
        n150 = Bundle(w289, w288, w287, w286, w282, "Measurement"=w281) -> (w306:T9)  [unwired: 1 in]
        n151 = Unbundle(w306) -> (w219:dbl, w213:dbl, w208:dbl, w203:dbl, w198:dbl, "Measurement"=w222:dbl)
        n152 = Unbundle(w306) -> (w304:dbl, w285:dbl, w284:dbl, w283:dbl, w305:dbl, "Measurement"=w271:dbl)
        n153 = Format Into String(format string="%08d  %8.2e %12g %14.5e %12.4e %12.4e  %12.4e %12.4e  %12.4e  %12g \\n", initial string=w348, w345, w305, w304, w285, w284, w283, w271, w182, w181, w180) -> ()  [unwired: 1 in, 2 out]
        n154 = Multiply(x=w222, y="2000") -> (x*y=w220:dbl)
        n155 = Multiply(x=w213, y="DAQ A1") -> (x*y=w214:dbl)
        n156 = Multiply(x=w219, y="DAQ A0") -> (x*y=w218:dbl)
        n157 = Multiply(x="DAQ A2", y=w208) -> (x*y=w209:dbl)
        n158 = Multiply(x=w198, y="DAQ A4") -> (x*y=w199:dbl)
        n159 = Multiply(x=w203, y="DAQ A3") -> (x*y=w204:dbl)
        n160 = Build Array (concatenate)(w453, w220) -> (w327:dbl[])
        n161 = Build Array (concatenate)(w333, w218) -> (w326:dbl[])
        n162 = Build Array (concatenate)(w332, w214) -> (w325:dbl[])
        n163 = Build Array (concatenate)(w331, w209) -> (w324:dbl[])
        n164 = Build Array (concatenate)(w442, w204) -> (w323:dbl[])
        n165 = Build Array (concatenate)(w278, w199) -> (w277:dbl[])
        n166 = Bundle(w329, w328, w327, w326, w325, w324, w323, w277, w280, w279) -> (w316:T10)  [unwired: 1 in]
        n167 = Unbundle(w316) -> (w228:dbl[], w186:dbl[], w225:dbl[], w216:dbl[], w211:dbl[], w206:dbl[], w201:dbl[], w195:dbl[], w191:dbl[], w185:dbl[])
        n168 = Bundle(w186, w228) -> (w229:cluster{dbl[], dbl[]})  [unwired: 1 in]
        n169 = Bundle(w186, w225) -> (w224:cluster{dbl[], dbl[]})  [unwired: 1 in]
        n170 = Bundle(w186, w216) -> (w215:cluster{dbl[], dbl[]})  [unwired: 1 in]
        n171 = Bundle(w186, w211) -> (w210:cluster{dbl[], dbl[]})  [unwired: 1 in]
        n172 = Bundle(w186, w201) -> (w200:cluster{dbl[], dbl[]})  [unwired: 1 in]
        n173 = Bundle(w186, w206) -> (w205:cluster{dbl[], dbl[]})  [unwired: 1 in]
        n174 = Bundle(w186, w195) -> (w196:cluster{dbl[], dbl[]})  [unwired: 1 in]
        n175 = Bundle(w186, w191) -> (w190:cluster{dbl[], dbl[]})  [unwired: 1 in]
        n176 = Bundle(w186, w185) -> (w184:cluster{dbl[], dbl[]})  [unwired: 1 in]
        n177 = Build Array(w229, w224, w215, w210, w205, w200, w196, w190, w184) -> (→"TIME GRAPH":cluster{dbl[], dbl[]}[])
        n178 = Unbundle(w316) -> (w315:dbl[], w314:dbl[], w313:dbl[], w312:dbl[], w311:dbl[], w310:dbl[], w309:dbl[], w308:dbl[], w272:dbl[])  [unwired: 1 out]
        n179 = case shown="\"V, Lock-In X\"" "X-Axis" {
          tunnel: [w457 w483 w502 w514 w540 w559 w578 w587 w606] -> w307
          tunnel: w315 -> [w454 w482 w501 w521 w539 w558 w576 w595 w614]
          tunnel: w314 -> [w471 w473 w500 w520 w538 w557 w575 w594 w613]
          tunnel: w313 -> [w470 w481 w492 w519 w537 w556 w574 w593 w612]
          tunnel: w312 -> [w469 w480 w499 w511 w536 w555 w573 w592 w611]
          tunnel: w311 -> [w468 w479 w498 w518 w530 w554 w572 w591 w610]
          tunnel: w310 -> [w467 w478 w497 w517 w535 w549 w571 w590 w609]
          tunnel: w309 -> [w466 w477 w496 w516 w534 w553 w577 w589 w608]
          tunnel: w308 -> [w465 w476 w495 w515 w533 w552 w570 w596 w607]
          tunnel: w272 -> [w455 w474 w493 w512 w531 w550 w569 w588 w615]
          frame "I, Keithley 6221", Default {
            n180 = property on="MULTIPLE GRAPHS" class="XYGraph (strict)"("XScale.NameLbl.Text"="Keithley 6221, mA" ("X Scale.Name Label.Text")) -> ()  [unwired: 2 in, 2 out]
            n181 = Bundle(w454, w471) -> (w464:cluster{dbl[], dbl[]})  [unwired: 1 in]
            n182 = Bundle(w454, w470) -> (w463:cluster{dbl[], dbl[]})  [unwired: 1 in]
            n183 = Bundle(w454, w469) -> (w462:cluster{dbl[], dbl[]})  [unwired: 1 in]
            n184 = Bundle(w454, w468) -> (w461:cluster{dbl[], dbl[]})  [unwired: 1 in]
            n185 = Bundle(w454, w467) -> (w460:cluster{dbl[], dbl[]})  [unwired: 1 in]
            n186 = Bundle(w454, w466) -> (w459:cluster{dbl[], dbl[]})  [unwired: 1 in]
            n187 = Bundle(w454, w465) -> (w458:cluster{dbl[], dbl[]})  [unwired: 1 in]
            n188 = Bundle(w454, w455) -> (w456:cluster{dbl[], dbl[]})  [unwired: 1 in]
            n189 = Build Array(w464, w463, w462, w461, w460, w459, w458, w456) -> (w457:cluster{dbl[], dbl[]}[])
          }
          frame "V, Keithley 2000" {
            n190 = property on="MULTIPLE GRAPHS" class="XYGraph (strict)"("XScale.NameLbl.Text"="Keithley 2000, V" ("X Scale.Name Label.Text")) -> ()  [unwired: 2 in, 2 out]
            n191 = Bundle(w473, w482) -> (w490:cluster{dbl[], dbl[]})  [unwired: 1 in]
            n192 = Bundle(w473, w481) -> (w489:cluster{dbl[], dbl[]})  [unwired: 1 in]
            n193 = Bundle(w473, w480) -> (w488:cluster{dbl[], dbl[]})  [unwired: 1 in]
            n194 = Bundle(w473, w479) -> (w487:cluster{dbl[], dbl[]})  [unwired: 1 in]
            n195 = Bundle(w473, w478) -> (w486:cluster{dbl[], dbl[]})  [unwired: 1 in]
            n196 = Bundle(w473, w477) -> (w485:cluster{dbl[], dbl[]})  [unwired: 1 in]
            n197 = Bundle(w473, w476) -> (w484:cluster{dbl[], dbl[]})  [unwired: 1 in]
            n198 = Bundle(w473, w474) -> (w475:cluster{dbl[], dbl[]})  [unwired: 1 in]
            n199 = Build Array(w490, w489, w488, w487, w486, w485, w484, w475) -> (w483:cluster{dbl[], dbl[]}[])
          }
          frame "V, Keithley DAQ A0" {
            n200 = property on="MULTIPLE GRAPHS" class="XYGraph (strict)"("XScale.NameLbl.Text"="Keithley DAQ A0, V" ("X Scale.Name Label.Text")) -> ()  [unwired: 2 in, 2 out]
            n201 = Bundle(w492, w493) -> (w494:cluster{dbl[], dbl[]})  [unwired: 1 in]
            n202 = Bundle(w492, w501) -> (w509:cluster{dbl[], dbl[]})  [unwired: 1 in]
            n203 = Bundle(w492, w500) -> (w508:cluster{dbl[], dbl[]})  [unwired: 1 in]
            n204 = Bundle(w492, w499) -> (w507:cluster{dbl[], dbl[]})  [unwired: 1 in]
            n205 = Bundle(w492, w498) -> (w506:cluster{dbl[], dbl[]})  [unwired: 1 in]
            n206 = Bundle(w492, w497) -> (w505:cluster{dbl[], dbl[]})  [unwired: 1 in]
            n207 = Bundle(w492, w496) -> (w504:cluster{dbl[], dbl[]})  [unwired: 1 in]
            n208 = Bundle(w492, w495) -> (w503:cluster{dbl[], dbl[]})  [unwired: 1 in]
            n209 = Build Array(w509, w508, w507, w506, w505, w504, w503, w494) -> (w502:cluster{dbl[], dbl[]}[])
          }
          frame "V, Keithley DAQ A1" {
            n210 = property on="MULTIPLE GRAPHS" class="XYGraph (strict)"("XScale.NameLbl.Text"="Keithley DAQ A1, V" ("X Scale.Name Label.Text")) -> ()  [unwired: 2 in, 2 out]
            n211 = Bundle(w511, w521) -> (w523:cluster{dbl[], dbl[]})  [unwired: 1 in]
            n212 = Bundle(w511, w520) -> (w524:cluster{dbl[], dbl[]})  [unwired: 1 in]
            n213 = Bundle(w511, w519) -> (w525:cluster{dbl[], dbl[]})  [unwired: 1 in]
            n214 = Bundle(w511, w518) -> (w526:cluster{dbl[], dbl[]})  [unwired: 1 in]
            n215 = Bundle(w511, w517) -> (w527:cluster{dbl[], dbl[]})  [unwired: 1 in]
            n216 = Bundle(w511, w516) -> (w528:cluster{dbl[], dbl[]})  [unwired: 1 in]
            n217 = Bundle(w511, w515) -> (w529:cluster{dbl[], dbl[]})  [unwired: 1 in]
            n218 = Bundle(w511, w512) -> (w513:cluster{dbl[], dbl[]})  [unwired: 1 in]
            n219 = Build Array(w523, w524, w525, w526, w527, w528, w529, w513) -> (w514:cluster{dbl[], dbl[]}[])
          }
          frame "V, Keithley DAQ A2" {
            n220 = property on="MULTIPLE GRAPHS" class="XYGraph (strict)"("XScale.NameLbl.Text"="Keithley DAQ A2, V" ("X Scale.Name Label.Text")) -> ()  [unwired: 2 in, 2 out]
            n221 = Bundle(w530, w539) -> (w541:cluster{dbl[], dbl[]})  [unwired: 1 in]
            n222 = Bundle(w530, w538) -> (w542:cluster{dbl[], dbl[]})  [unwired: 1 in]
            n223 = Bundle(w530, w537) -> (w543:cluster{dbl[], dbl[]})  [unwired: 1 in]
            n224 = Bundle(w530, w536) -> (w544:cluster{dbl[], dbl[]})  [unwired: 1 in]
            n225 = Bundle(w530, w535) -> (w545:cluster{dbl[], dbl[]})  [unwired: 1 in]
            n226 = Bundle(w530, w534) -> (w546:cluster{dbl[], dbl[]})  [unwired: 1 in]
            n227 = Bundle(w530, w533) -> (w547:cluster{dbl[], dbl[]})  [unwired: 1 in]
            n228 = Bundle(w530, w531) -> (w532:cluster{dbl[], dbl[]})  [unwired: 1 in]
            n229 = Build Array(w541, w542, w543, w544, w545, w546, w547, w532) -> (w540:cluster{dbl[], dbl[]}[])
          }
          frame "V, Keithley DAQ A3" {
            n230 = property on="MULTIPLE GRAPHS" class="XYGraph (strict)"("XScale.NameLbl.Text"="Keithley DAQ A3, V" ("X Scale.Name Label.Text")) -> ()  [unwired: 2 in, 2 out]
            n231 = Bundle(w549, w558) -> (w560:cluster{dbl[], dbl[]})  [unwired: 1 in]
            n232 = Bundle(w549, w557) -> (w561:cluster{dbl[], dbl[]})  [unwired: 1 in]
            n233 = Bundle(w549, w556) -> (w562:cluster{dbl[], dbl[]})  [unwired: 1 in]
            n234 = Bundle(w549, w555) -> (w563:cluster{dbl[], dbl[]})  [unwired: 1 in]
            n235 = Bundle(w549, w554) -> (w564:cluster{dbl[], dbl[]})  [unwired: 1 in]
            n236 = Bundle(w549, w553) -> (w565:cluster{dbl[], dbl[]})  [unwired: 1 in]
            n237 = Bundle(w549, w552) -> (w566:cluster{dbl[], dbl[]})  [unwired: 1 in]
            n238 = Bundle(w549, w550) -> (w551:cluster{dbl[], dbl[]})  [unwired: 1 in]
            n239 = Build Array(w560, w561, w562, w563, w564, w565, w566, w551) -> (w559:cluster{dbl[], dbl[]}[])
          }
          frame "V, Keithley DAQ A4" {
            n240 = property on="MULTIPLE GRAPHS" class="XYGraph (strict)"("XScale.NameLbl.Text"="Keithley DAQ A4, V" ("X Scale.Name Label.Text")) -> ()  [unwired: 2 in, 2 out]
            n241 = Bundle(w577, w576) -> (w580:cluster{dbl[], dbl[]})  [unwired: 1 in]
            n242 = Bundle(w577, w575) -> (w581:cluster{dbl[], dbl[]})  [unwired: 1 in]
            n243 = Bundle(w577, w574) -> (w582:cluster{dbl[], dbl[]})  [unwired: 1 in]
            n244 = Bundle(w577, w573) -> (w583:cluster{dbl[], dbl[]})  [unwired: 1 in]
            n245 = Bundle(w577, w572) -> (w584:cluster{dbl[], dbl[]})  [unwired: 1 in]
            n246 = Bundle(w577, w571) -> (w585:cluster{dbl[], dbl[]})  [unwired: 1 in]
            n247 = Bundle(w577, w570) -> (w586:cluster{dbl[], dbl[]})  [unwired: 1 in]
            n248 = Bundle(w577, w569) -> (w579:cluster{dbl[], dbl[]})  [unwired: 1 in]
            n249 = Build Array(w580, w581, w582, w583, w584, w585, w586, w579) -> (w578:cluster{dbl[], dbl[]}[])
          }
          frame "V, Lock-In X" {
            n250 = property on="MULTIPLE GRAPHS" class="XYGraph (strict)"("XScale.NameLbl.Text"="Lock-In X, V" ("X Scale.Name Label.Text")) -> ()  [unwired: 2 in, 2 out]
            n251 = Bundle(w596, w595) -> (w598:cluster{dbl[], dbl[]})  [unwired: 1 in]
            n252 = Bundle(w596, w594) -> (w599:cluster{dbl[], dbl[]})  [unwired: 1 in]
            n253 = Bundle(w596, w593) -> (w600:cluster{dbl[], dbl[]})  [unwired: 1 in]
            n254 = Bundle(w596, w592) -> (w601:cluster{dbl[], dbl[]})  [unwired: 1 in]
            n255 = Bundle(w596, w591) -> (w602:cluster{dbl[], dbl[]})  [unwired: 1 in]
            n256 = Bundle(w596, w590) -> (w603:cluster{dbl[], dbl[]})  [unwired: 1 in]
            n257 = Bundle(w596, w589) -> (w604:cluster{dbl[], dbl[]})  [unwired: 1 in]
            n258 = Bundle(w596, w588) -> (w597:cluster{dbl[], dbl[]})  [unwired: 1 in]
            n259 = Build Array(w598, w599, w600, w601, w602, w603, w604, w597) -> (w587:cluster{dbl[], dbl[]}[])
          }
          frame "V, Lock-In Y" {
            n260 = property on="MULTIPLE GRAPHS" class="XYGraph (strict)"("XScale.NameLbl.Text"="Lock-In Y, V" ("X Scale.Name Label.Text")) -> ()  [unwired: 2 in, 2 out]
            n261 = Bundle(w615, w614) -> (w623:cluster{dbl[], dbl[]})  [unwired: 1 in]
            n262 = Bundle(w615, w613) -> (w622:cluster{dbl[], dbl[]})  [unwired: 1 in]
            n263 = Bundle(w615, w612) -> (w621:cluster{dbl[], dbl[]})  [unwired: 1 in]
            n264 = Bundle(w615, w611) -> (w620:cluster{dbl[], dbl[]})  [unwired: 1 in]
            n265 = Bundle(w615, w610) -> (w619:cluster{dbl[], dbl[]})  [unwired: 1 in]
            n266 = Bundle(w615, w609) -> (w618:cluster{dbl[], dbl[]})  [unwired: 1 in]
            n267 = Bundle(w615, w608) -> (w617:cluster{dbl[], dbl[]})  [unwired: 1 in]
            n268 = Bundle(w615, w607) -> (w616:cluster{dbl[], dbl[]})  [unwired: 1 in]
            n269 = Build Array(w623, w622, w621, w620, w619, w618, w617, w616) -> (w606:cluster{dbl[], dbl[]}[])
          }
        }
        "MULTIPLE GRAPHS" <- w307
        n270 = Unbundle(w316) -> (w322:dbl[], w321:dbl[], w320:dbl[], w319:dbl[], w318:dbl[], w317:dbl[], w273:dbl[], w274:dbl[], w275:dbl[], w276:dbl[])
        "2000" <- w433
        "DAQ A0" <- w289
        "DAQ A1" <- w288
        "DAQ A2" <- w287
        "DAQ A3" <- w286
        "DAQ A4" <- w282
      }
    }
    frame #3 {
      # "Closing instrumental \nconnections"
      n271 = Unbundle(w883) -> ("Task out"=w882:i32, "error out"=w881:errorcluster)
      n272 = call <instrlib>:"Close.vi"("VISA resource name"=w888, "error in (no error)"=w889) -> ()  [unwired: 17 in, 1 out]
      n273 = call "SR51XX Close"("error in (no error)"=w884, "VISA session"=w885) -> ()  [unwired: 1 out]
      n274 = call <instrlib>:"Close.vi"("VISA resource name"=w886, "error in (no error)"=w887) -> ()  [unwired: 13 in, 1 out]
      n275 = call <userlib>:"DtOLCloseTask.vi"("Error in"=w881, "Task in"=w882) -> ("Error Out"=w890:errorcluster)  [unwired: 9 in]
      n276 = call <vilib>:"Simple Error Handler.vi"("error in (no error)"=w890) -> ()  [unwired: 4 in, 5 out]
    }
  }
